vi "U8 Counter.vi"(10 "reset (F)":bool, 11 "increment":bool) -> (3 "count":u8)   [LabVIEW 2013, in "I2S-TDM.lvlib"]
uses:
  I2S-TDM.lvlib
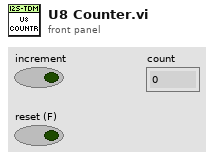
[diagram p1: front panel]
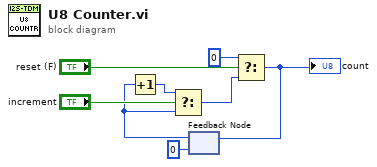
[diagram p0: block diagram]
diagram:
  n1 = feedback #1(u8 0) -> (w2:u8)
  n2 = Increment(x=w2) -> (x+1=w1:u8)
  n3 = Select(t=w1, s="increment", f=w2) -> (s? t:f=w7:u8)
  n4 = Select(t=u8 0, s="reset (F)", f=w7) -> (s? t:f=w8:u8)
  "count" <- w8
  n5 = feedback-in #1(w8) -> ()
